vi "New Node.vi"(8 "error in (no error)":errorcluster, 9 "Display Name":string, 10 "UID":string, 11 "UA Server in":refnum<class "UA Server.lvclass">) -> (0 "error out":errorcluster, 2 "Generic Node out":refnum<class "Generic Node.lvclass">, 3 "UA Server out":refnum<class "UA Server.lvclass">)   [LabVIEW 2017, in "opcua.lvlib" / "Browser Core.lvlib" / "UA Server.lvclass"]
doc: "Create new Node Class from UID Input"
uses:
  UA Server.lvclass
  Node Classes/Generic Node/Generic Node.lvclass
  Node Classes/UA Node/UA Node.lvclass
  Node Classes/UA Node/Node Class.ctl
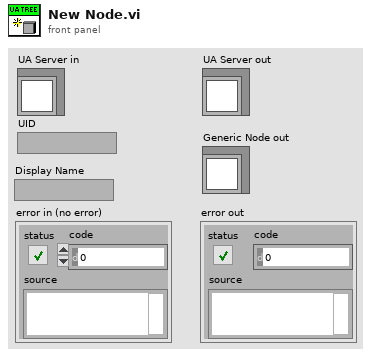
[diagram p1: front panel]
types:
  T1 = cluster{"name":string, "node class":u16, "data type":u16, "access":enum16{"Null", "Read", "Write", "Read&Write"}, "description":string}
  T2 = typedef "opcua.lvlib/Browser Core.lvlib/UA Node.lvclass/Node Class.ctl" = u16
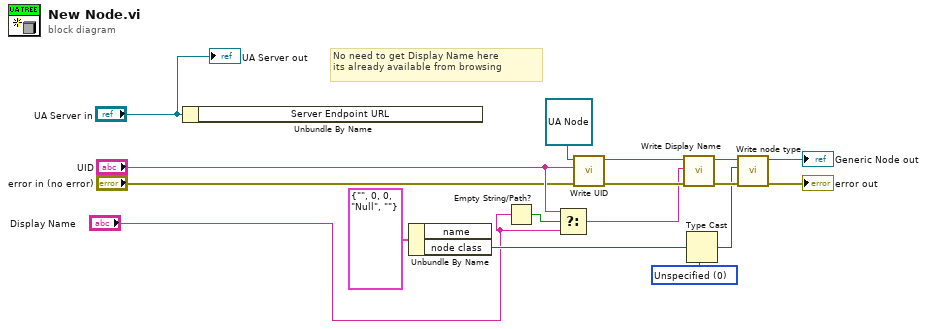
[diagram p0: block diagram]
diagram:
  w8 = T2 0 items=["Unspecified"=0, "Object"=1, "Variable"=2, "Method"=4, "Object Type"=8, "Variable Type"=16, "Reference Type"=32, "Data Type"=64, "View"=128] ("node class")
  # "No need to get Display Name here\nits already available from browsing"
  n1 = Unbundle By Name("UA Server in") -> ()  [unwired: 1 out]
  n2 = Unbundle By Name(T1 {"name"="", "node class"=0, "data type"=0, "access"=enum."Null", "description"=""} ("input cluster")) -> ("node class"=w2:u16)  [unwired: 1 out]
  n3 = Empty String/Path?(string/path="Display Name") -> (empty?=w7:bool)
  n4 = Select(t="UID", s=w7, f="Display Name") -> (s? t:f=w6:string)
  n5 = call "Write UID.vi"("error in (no error)"="error in (no error)", "UID"="UID", "Generic Node in"=refnum<class "UA Node.lvclass"> refnum ("Browser Core.lvlib:UA Node.lvclass")) -> ("error out"=w15:errorcluster, "Generic Node out"=w16:refnum<class "UA Node.lvclass">)  [unwired: 7 in]
  n6 = call "Write Display Name.vi"("error in (no error)"=w15, "Display Name"=w6, "Generic Node in"=w16) -> ("error out"=w13:errorcluster, "Generic Node out"=w14:refnum<class "UA Node.lvclass">)  [unwired: 7 in]
  n7 = Type Cast(type=w8, x=w2) -> (*(type *) &x=w9:T2)
  n8 = call "Write node type.vi"("error in (no error)"=w13, "node class"=w9, "UA Node in"=w14) -> ("error out"=→"error out":errorcluster, "UA Node out"=→"Generic Node out":refnum<class "UA Node.lvclass">)  [unwired: 7 in]
  "UA Server out" <- "UA Server in"
